vi "Concept of LOG_fpga_dsp48e.vi"() -> ()   [LabVIEW 2011]
uses:
  <vilib>/rvi/FXPMathLib/FxpInterpret/XNode/nifxpmath_Interpret.xnode
panel:
  in  "LUT":fxp<+/-,20,8>[](array[numeric])=[-128.0, -27.0927734375, -24.08251953125, -22.321533203125, -21.072021484375, -20.10302734375, -19.311279296875, -18.6416015625, -18.061767578125, -17.55029296875, -17.0927734375, -16.6787109375, -16.30078125, -15.953369140625, -15.63134765625, -15.331787109375, -15.051513671875, -14.788330078125, -14.5400390625, -14.30517578125, -14.08251953125, -13.87060546875, -13.66845703125, -13.475341796875, -13.29052734375, -13.11328125, -12.94287109375, -12.779052734375, -12.62109375, -12.46875, -12.321533203125, -12.17919921875, -12.041259765625, -11.907470703125, -11.77783203125, -11.652099609375, -11.52978515625, -11.41064453125, -11.294921875, -11.18212890625, -11.072021484375, -10.96484375, -10.860107421875, -10.758056640625, -10.658203125, -10.560546875, -10.465087890625, -10.371826171875, -10.2802734375, -10.190673828125, -10.10302734375, -10.01708984375, -9.9326171875, -9.849853515625, -9.768798828125, -9.68896484375, -9.61083984375, -9.533935546875, -9.45849609375, -9.38427734375, -9.311279296875, -9.239501953125, -9.168701171875, -9.099365234375, -9.031005859375, -8.963623046875, -8.897216796875, -8.83203125, -8.767578125, -8.7041015625, -8.6416015625, -8.580078125, -8.519287109375, -8.45947265625, -8.400390625, -8.342041015625, -8.28466796875, -8.227783203125, -8.171875, -8.116455078125, -8.061767578125, -8.0078125, -7.95458984375, -7.90185546875, -7.849853515625, -7.798583984375, -7.747802734375, -7.697509765625, -7.64794921875, -7.598876953125, -7.55029296875, -7.502197265625, -7.454833984375, -7.407958984375, -7.361328125, -7.3154296875, -7.27001953125, -7.22509765625, -7.180419921875, -7.13623046875, -7.0927734375, -7.049560546875, -7.006591796875, -6.96435546875, -6.92236328125, -6.880859375, -6.839599609375, -6.798828125, -6.758544921875, -6.718505859375, -6.6787109375, -6.639404296875, -6.6005859375, -6.56201171875, -6.523681640625, -6.48583984375, -6.447998046875, -6.410888671875, -6.373779296875, -6.337158203125, -6.30078125, -6.264892578125, -6.22900390625, -6.193603515625, -6.158447265625, -6.12353515625, -6.089111328125, -6.0546875, -6.0205078125, -5.98681640625, -5.953369140625, -5.919921875, -5.886962890625, -5.854248046875, -5.821533203125, -5.789306640625, -5.75732421875, -5.7255859375, -5.69384765625, -5.66259765625, -5.63134765625, -5.6005859375, -5.56982421875, -5.539306640625, -5.509033203125, -5.47900390625, -5.44921875, -5.41943359375, -5.39013671875, -5.36083984375, -5.331787109375, -5.302978515625, -5.274169921875, -5.245849609375, -5.217529296875, -5.189453125, -5.161376953125, -5.1337890625, -5.106201171875, -5.07861328125, -5.051513671875, -5.0244140625, -4.99755859375, -4.970703125, -4.9443359375, -4.91796875, -4.8916015625, -4.865478515625, -4.839599609375, -4.813720703125, -4.788330078125, -4.7626953125, -4.7373046875, -4.712158203125, -4.687255859375, -4.662353515625, -4.637451171875, -4.613037109375, -4.58837890625, -4.564208984375, -4.5400390625, -4.515869140625, -4.491943359375, -4.46826171875, -4.444580078125, -4.4208984375, -4.3974609375, -4.374267578125, -4.35107421875, -4.328125, -4.30517578125, -4.282470703125, -4.259765625, -4.237060546875, -4.214599609375, -4.1923828125, -4.170166015625, -4.14794921875, -4.1259765625, -4.104248046875, -4.08251953125, -4.060791015625, -4.039306640625, -4.017822265625, -3.996337890625, -3.97509765625, -3.9541015625, -3.93310546875, -3.912109375, -3.891357421875, -3.87060546875, -3.849853515625, -3.829345703125, -3.808837890625, -3.78857421875, -3.768310546875, -3.748046875, -3.72802734375, -3.708251953125, -3.688232421875, -3.66845703125, -3.648681640625, -3.629150390625, -3.609619140625, -3.59033203125, -3.57080078125, -3.551513671875, -3.532470703125, -3.513427734375, -3.494384765625, -3.475341796875, -3.45654296875, -3.437744140625, -3.419189453125, -3.400634765625, -3.382080078125, -3.363525390625, -3.34521484375, -3.326904296875, -3.308837890625, -3.29052734375, -3.2724609375, -3.254638671875, -3.236572265625, -3.21875, -3.200927734375, -3.183349609375, -3.165771484375, -3.148193359375, -3.130615234375, -3.11328125, -3.095947265625, -3.07861328125, -3.0615234375, -3.04443359375, -3.02734375, -3.01025390625, -2.993408203125, -2.9765625, -2.959716796875, -2.94287109375, -2.92626953125, -2.90966796875, -2.89306640625, -2.876708984375, -2.8603515625, -2.843994140625, -2.82763671875, -2.811279296875, -2.795166015625, -2.779052734375, -2.762939453125, -2.7470703125, -2.73095703125, -2.715087890625, -2.699462890625, -2.68359375, -2.66796875, -2.65234375, -2.63671875, -2.62109375, -2.605712890625, -2.590087890625, -2.574951171875, -2.5595703125, -2.544189453125, -2.529052734375, -2.513916015625, -2.498779296875, -2.483642578125, -2.46875, -2.453857421875, -2.43896484375, -2.424072265625, -2.4091796875, -2.39453125, -2.3798828125, -2.365234375, -2.3505859375, -2.3359375, -2.321533203125, -2.30712890625, -2.292724609375, -2.2783203125, -2.263916015625, -2.249755859375, -2.235595703125, -2.221435546875, -2.207275390625, -2.193115234375, -2.17919921875, -2.1650390625, -2.151123046875, -2.13720703125, -2.123291015625, -2.109619140625, -2.095947265625, -2.08203125, -2.068359375, -2.0546875, -2.041259765625, -2.027587890625, -2.01416015625, -2.000732421875, -1.9873046875, -1.973876953125, -1.96044921875, -1.947265625, -1.93408203125, -1.920654296875, -1.907470703125, -1.89453125, -1.88134765625, -1.8681640625, -1.855224609375, -1.84228515625, -1.829345703125, -1.81640625, -1.803466796875, -1.790771484375, -1.77783203125, -1.76513671875, -1.75244140625, -1.73974609375, -1.72705078125, -1.714599609375, -1.701904296875, -1.689453125, -1.677001953125, -1.66455078125, -1.652099609375, -1.6396484375, -1.627197265625, -1.614990234375, -1.602783203125, -1.59033203125, -1.578125, -1.56591796875, -1.553955078125, -1.541748046875, -1.52978515625, -1.517578125, -1.505615234375, -1.49365234375, -1.481689453125, -1.4697265625, -1.4580078125, -1.446044921875, -1.434326171875, -1.42236328125, -1.41064453125, -1.39892578125, -1.38720703125, -1.375732421875, -1.364013671875, -1.352294921875, -1.3408203125, -1.329345703125, -1.31787109375, -1.306396484375, -1.294921875, -1.283447265625, -1.27197265625, -1.2607421875, -1.249267578125, -1.238037109375, -1.226806640625, -1.215576171875, -1.204345703125, -1.193115234375, -1.18212890625, -1.1708984375, -1.159912109375, -1.148681640625, -1.1376953125, -1.126708984375, -1.11572265625, -1.104736328125, -1.09375, -1.0830078125, -1.072021484375, -1.061279296875, -1.050537109375, -1.03955078125, -1.02880859375, -1.01806640625, -1.00732421875, -0.996826171875, -0.986083984375, -0.9755859375, -0.96484375, -0.954345703125, -0.94384765625, -0.93310546875, -0.922607421875, -0.912109375, -0.90185546875, -0.891357421875, -0.880859375, -0.87060546875, -0.860107421875, -0.849853515625, -0.839599609375, -0.829345703125, -0.819091796875, -0.808837890625, -0.798583984375, -0.788330078125, -0.7783203125, -0.76806640625, -0.758056640625, -0.748046875, -0.73779296875, -0.727783203125, -0.7177734375, -0.707763671875, -0.69775390625, -0.68798828125, -0.677978515625, -0.66796875, -0.658203125, -0.648193359375, -0.638427734375, -0.628662109375, -0.618896484375, -0.609130859375, -0.599365234375, -0.589599609375, -0.579833984375, -0.5703125, -0.560546875, -0.551025390625, -0.541259765625, -0.53173828125, -0.522216796875, -0.5126953125, -0.5029296875, -0.49365234375, -0.484130859375, -0.474609375, -0.465087890625, -0.455810546875, -0.4462890625, -0.43701171875, -0.427490234375, -0.418212890625, -0.408935546875, -0.3994140625, -0.39013671875, -0.380859375, -0.371826171875, -0.362548828125, -0.353271484375, -0.343994140625, -0.3349609375, -0.32568359375, -0.316650390625, -0.3076171875, -0.29833984375, -0.289306640625, -0.2802734375, -0.271240234375, -0.26220703125, -0.253173828125, -0.244140625, -0.2353515625, -0.226318359375, -0.217529296875, -0.20849609375, -0.19970703125, -0.190673828125, -0.181884765625, -0.173095703125, -0.164306640625, -0.155517578125, -0.146728515625, -0.137939453125, -0.129150390625, -0.120361328125, -0.111572265625, -0.10302734375, -0.09423828125, -0.085693359375, -0.076904296875, -0.068359375, -0.059814453125, -0.05126953125, -0.042724609375, -0.0341796875, -0.025634765625, -0.01708984375, -0.008544921875] format="%.15g"
  out "Truncated Address":u16
  out "Mantissa (M)":u32
  out "Exponent (-N)":i8
  out "LUT calculation":fxp<+/-,33,16> format="%.22g"
  in  "Input Number (1.32)":fxp<+,32,1>
  # "Output"
  # "Test Cases for Magnitude\n2.32831E-10\n1\n0\n0.567893"
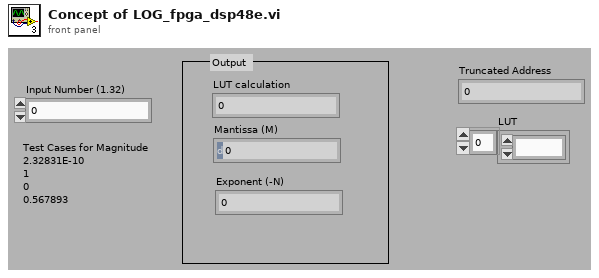
[diagram p1: front panel]
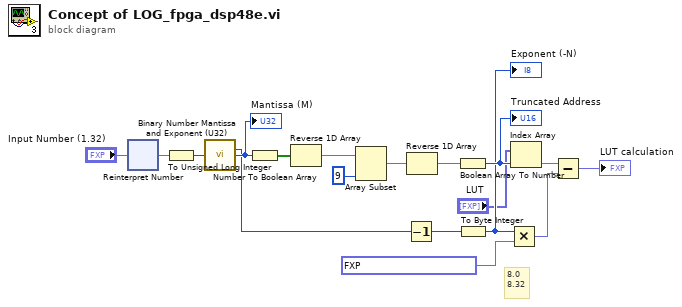
[diagram p0: block diagram]
diagram:
  # "8.0\n8.32"
  n1 = xnode "Reinterpret Number"("x"="Input Number (1.32)") -> ("y"=w18:fxp<+,32,32>)
  n2 = To Unsigned Long Integer(number=w18) -> (unsigned 32bit integer=w17:u32)
  n3 = call <userlib>:"Binary Number Mantissa and Exponent (U32).vi"("Binary Number"=w17) -> ("Exponent (-N)"=w7:i8, "Mantissa (M)"=w8:u32)  [unwired: 12 in, 1 out]
  "Mantissa (M)" <- w8
  n4 = Number To Boolean Array(number=w8) -> (Boolean array=w15:bool[])
  n5 = Reverse 1D Array(array=w15) -> (reversed array=w14:bool[])
  n6 = Array Subset(array=w14, length=9) -> (w12:bool[])  [unwired: 1 in]
  n7 = Decrement(x=w7) -> (x-1=w3:i8)
  n8 = Reverse 1D Array(array=w12) -> (reversed array=w11:bool[])
  n9 = Boolean Array To Number(Boolean array=w11) -> (number=w13:u16)
  "Truncated Address" <- w13
  n10 = To Byte Integer(number=w3) -> (8bit integer=w2:i8)
  "Exponent (-N)" <- w2
  n11 = Multiply(x=w2, y=fxp<+/-,25,8> 3.0102996826171875 ("fixed-point")) -> (x*y=w4:fxp<+/-,33,16>)
  n12 = Index Array(array="LUT", index=w13) -> (element=w10:fxp<+/-,20,8>)
  n13 = Subtract(x=w10, y=w4) -> (x-y=→"LUT calculation":fxp<+/-,33,16>)
